vi "RVHR Run MetaInfo.vi"(8 "error in (no error)":errorcluster, 10 "Run Info":T1 {"Date" format="%<%d/%m/%Y>T"}) -> (0 "error out":errorcluster, 2 "RVHR Info File":T2, 3 "Cancel?":bool)   [LabVIEW 2024]
uses:
  Buttons/OK.ctl
  Buttons/Cancel.ctl
  Controls/Sum File Cluster (RCA).ctl
  Controls/File Information CLuster.ctl
  Controls/Run Description.ctl
  Controls/Run information (YRCA).ctl
  Controls/System information (YRCA - Truncate).ctl
panel:
  in  "OK Button":T7
  in  "Cancel Button":T8
  in  "Ref Profile":string caption="Ref Profile:"
  in  "Company":string caption="Company:"
  in  "Location":string caption="Location:"
  in  "Operator":string caption="Operator:"
  in  "Date":timestamp caption="Date:" format="%<%d/%m/%Y>T"
  in  "Run End":dbl caption="Run End:" format="%.3f km"
  in  "Run Start":dbl caption="Run Start:" format="%.3f km"
  in  "Notes":string caption="Notes:"
  # "Enter Information for the Run:"
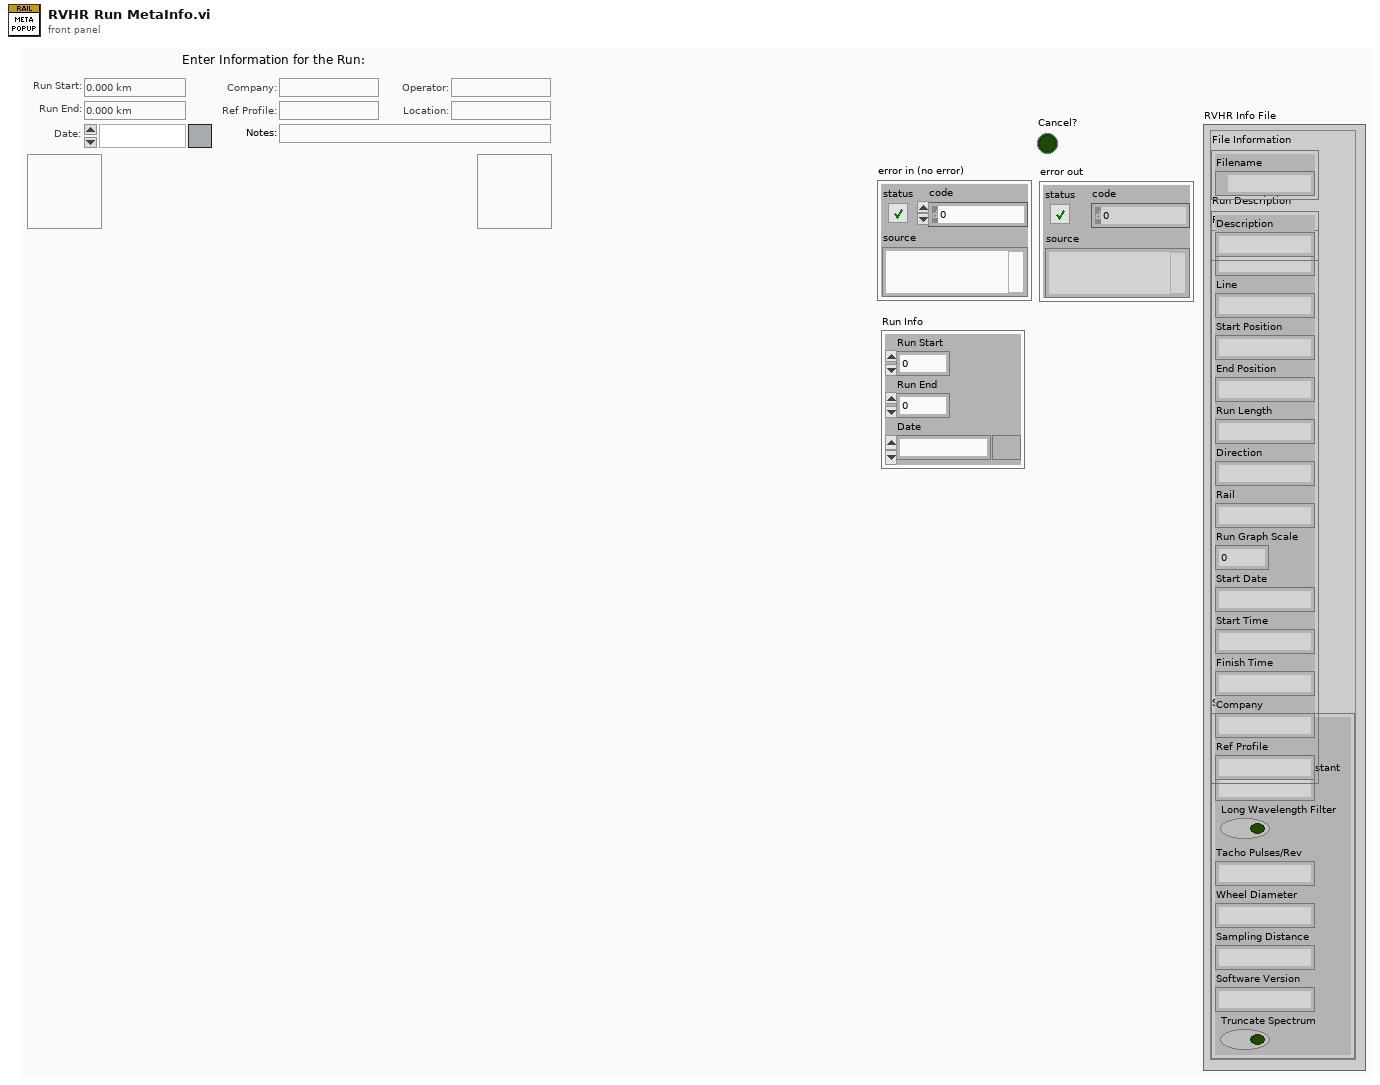
[diagram p1: front panel]
types:
  T1 = cluster{"Run Start":dbl, "Run End":dbl, "Date":timestamp}
  T2 = typedef "Sum File Cluster (RCA).ctl" = cluster{"File Information":T3, "Run Description":T4, "Run Information":T5, "System Information":T6}
  T3 = typedef "File Information CLuster.ctl" = cluster{"Filename":path}
  T4 = typedef "Run Description.ctl" = cluster{"Description":string}
  T5 = typedef "Run information (YRCA).ctl" = cluster{"Operator":string, "Line":string, "Start Position":string, "End Position":string, "Run Length":string, "Direction":string, "Rail":string, "Run Graph Scale":u16, "Start Date":string, "Start Time":string, "Finish Time":string, "Company":string, "Ref Profile":string}
  T6 = typedef "System information (YRCA - Truncate).ctl" = cluster{"Sensor Calibration":string, "Integrator Time Constant":string, "Long Wavelength Filter":bool, "Tacho Pulses/Rev":string, "Wheel Diameter":string, "Sampling Distance":string, "Software Version":string, "Truncate Spectrum":bool}
  T7 = typedef "OK.ctl" = bool
  T8 = typedef "Cancel.ctl" = bool
  T9 = enum8{"Enabled", "Disabled", "Disabled and Grayed Out"}
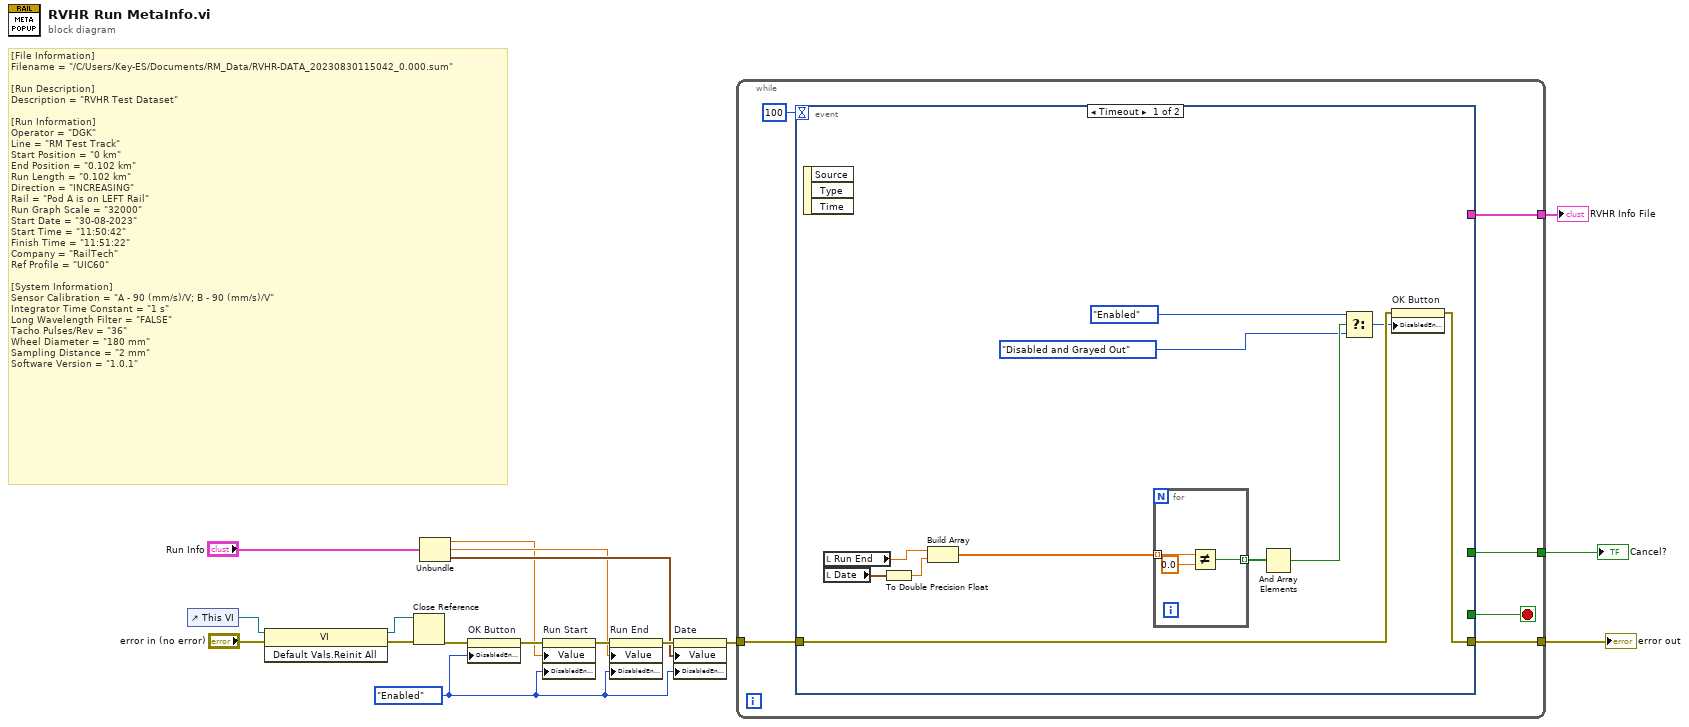
[diagram p0: block diagram]
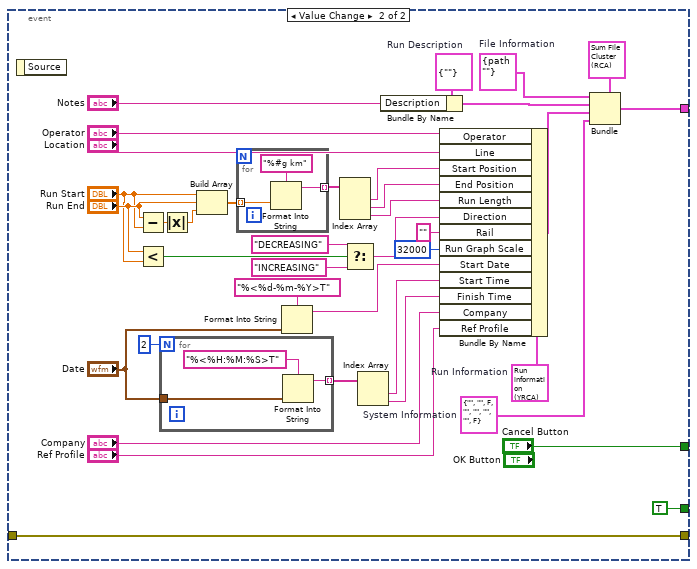
[diagram p2: hidden frame]
diagram:
  w1 = T9."Enabled" ("Disabled")
  # "[File Information]\nFilename = \"/C/Users/Key-ES/Documents/RM_Data/RVHR-DATA_20230830115042_0.000.sum\"\n\n[Run Description]\nDescription = \"RVHR Test Dataset\"\n\n[Run Information]\nOperator = \"DGK\"\nLine = \"RM Test Track\"\nStart Position = \"0 km\"\nEnd Position = \"0.102 km\"\nRun Length = \"0.102 km\"\nDirection = \"INCREASING\"\nRail = \"Pod A is on LEFT Rail\"\nRun Graph Scale = \"32000\"\nStart Date = \"30-08-2023\"\nStart Time = \"11:50:42\"\nFinish Time = \"11:51:22\"\nCompany = \"RailTech\"\nRef Profile = \"UIC60\"\n\n[System Information]\nSensor Calibration = \"A - 90 (mm/s)/V; B - 90 (mm/s)/V\"\nIntegrator Time Constant = \"1 s\"\nLong Wavelength Filter = \"FALSE\"\nTacho Pulses/Rev = \"36\"\nWheel Diameter = \"180 mm\"\nSampling Distance = \"2 mm\"\nSoftware Version = \"1.0.1\""
  n1 = control-ref of="This VI"() -> (w13:refnum<vi>)
  n2 = invoke class="VI" method="Default Vals.Reinit All"(reference=w13, error in="error in (no error)") -> (reference out=w12:refnum<vi>, error out=w14:errorcluster)  [unwired: 1 in, 1 out]
  n3 = Close Reference(reference=w12, error in (no error)=w14) -> (error out=w11:errorcluster)
  n4 = Unbundle("Run Info") -> ("Run Start"=w2:dbl, "Run End"=w3:dbl, "Date"=w4:timestamp)
  n5 = property on="OK Button" class="Bool"(error in=w11, "DisabledEnum"=w1) -> (error out=w6:errorcluster)  [unwired: 1 in, 1 out]
  n6 = property on="Run Start" class="DigNum (strict)"(error in=w6, "Value"=w2, "DisabledEnum"=w1) -> (error out=w9:errorcluster)  [unwired: 1 in, 1 out]
  n7 = property on="Run End" class="DigNum (strict)"(error in=w9, "Value"=w3, "DisabledEnum"=w1) -> (error out=w8:errorcluster)  [unwired: 1 in, 1 out]
  n8 = property on="Date" class="AbsTime (strict)"(error in=w8, "Value"=w4, "DisabledEnum"=w1) -> (error out=w7:errorcluster)  [unwired: 1 in, 1 out]
  n9 = while {
    tunnel: w7 -> [w23]
    tunnel: [w22] -> w16
    tunnel: [w21] -> w15
    tunnel: [w18] -> w10
    stop <- w20 stop-if-true
    n10 = event shown="[0] Timeout" {
      selector: _ -> [_ _]
      dyn-events: _ -> [_ _]
      timeout: 100 -> [_ _]
      tunnel: w23 -> [w29 w75]
      tunnel: [w28 w75] -> w22
      tunnel: [_ "Cancel Button"] -> w21
      tunnel: [_ TRUE] -> w20
      tunnel: [_ w38] -> w18
      event Timeout {
        n11 = event-data() -> ()  [unwired: 1 in, 3 out]
        n12 = local read "Run End"() -> (w33:dbl)
        n13 = local read "Date"() -> (w32:timestamp)
        n14 = To Double Precision Float(number=w32) -> (double precision float=w31:dbl)
        n15 = Build Array(w33, w31) -> (w34:dbl[])
        n16 = for {
          tunnel: w34 -> [w36] mode=indexing
          tunnel: [w35] -> w30 mode=indexing
          n17 = Not Equal?(x=w36, y=0.0) -> (x != y?=w35:bool)
        }
        n18 = And Array Elements(Boolean array=w30) -> (logical AND=w27:bool)
        n19 = Select(t=T9."Enabled", s=w27, f=T9."Disabled and Grayed Out" ("Disabled")) -> (s? t:f=w25:T9)
        n20 = property on="OK Button" class="Bool"(error in=w29, "DisabledEnum"=w25) -> (error out=w28:errorcluster)  [unwired: 1 in, 1 out]
      }
      event Value Change {
        w64 = T6 {"Sensor Calibration"="", "Integrator Time Constant"="", "Long Wavelength Filter"=FALSE, "Tacho Pulses/Rev"="", "Wheel Diameter"="", "Sampling Distance"="", "Software Version"="", "Truncate Spectrum"=FALSE}  # System Information
        w67 = T5 {"Operator"="", "Line"="", "Start Position"="", "End Position"="", "Run Length"="", "Direction"="", "Rail"="", "Run Graph Scale"=0, "Start Date"="", "Start Time"="", "Finish Time"="", "Company"="", "Ref Profile"=""}  # Run Information
        w69 = T3 {"Filename"=path ""}  # File Information
        w71 = T4 {"Description"=""}  # Run Description
        n21 = event-data() -> ()  [unwired: 1 in, 1 out]
        n22 = Subtract(x="Run End", y="Run Start") -> (x-y=w57:dbl)
        n23 = Less?(x="Run End", y="Run Start") -> (x < y?=w46:bool)
        n24 = for {
          N: 2 -> [_]
          tunnel: "Date" -> [w77]
          tunnel: [w76] -> w45 mode=indexing
          n25 = Format Into String(format string="%<%H:%M:%S>T", w77) -> (resulting string=w76:string)  [unwired: 2 in, 1 out]
        }
        n26 = Absolute Value(x=w57) -> (abs(x)=w58:dbl)
        n27 = Build Array("Run Start", "Run End", w58) -> (w56:dbl[])
        n28 = for {
          tunnel: w56 -> [w81] mode=indexing
          tunnel: [w79] -> w55 mode=indexing
          n29 = Format Into String(format string="%#g km", w81) -> (resulting string=w79:string)  [unwired: 2 in, 1 out]
        }
        n30 = Format Into String(format string="%<%d-%m-%Y>T", "Date") -> (resulting string=w41:string)  [unwired: 2 in, 1 out]
        n31 = Index Array(array=w55) -> (element #1=w54:string, element #2=w53:string, element #3=w52:string)  [unwired: 3 in]
        n32 = Select(t="DECREASING", s=w46, f="INCREASING") -> (s? t:f=w49:string)
        n33 = Index Array(array=w45) -> (element #1=w40:string, element #2=w39:string)  [unwired: 2 in]
        n34 = Bundle By Name(cluster=w71, "Description"="Notes") -> (w68:T4)
        n35 = Bundle By Name(cluster=w67, "Operator"="Operator", "Line"="Location", "Start Position"=w54, "End Position"=w53, "Run Length"=w52, "Direction"=w49, "Rail"="", "Run Graph Scale"=u16 32000, "Start Date"=w41, "Start Time"=w40, "Finish Time"=w39, "Company"="Company", "Ref Profile"="Ref Profile") -> (w65:T5)
        n36 = Bundle(cluster=T2 {"File Information"={"Filename"=path ""}, "Run Description"={"Description"=""}, "Run Information"={"Operator"="", "Line"="", "Start Position"="", "End Position"="", "Run Length"="", "Direction"="", "Rail"="", "Run Graph Scale"=0, "Start Date"="", "Start Time"="", "Finish Time"="", "Company"="", "Ref Profile"=""}, "System Information"={"Sensor Calibration"="", "Integrator Time Constant"="", "Long Wavelength Filter"=FALSE, "Tacho Pulses/Rev"="", "Wheel Diameter"="", "Sampling Distance"="", "Software Version"="", "Truncate Spectrum"=FALSE}} ("output cluster"), "File Information"=w69, "Run Description"=w68, "Run Information"=w65, "System Information"=w64) -> (w38:T2)
      }
    }
  }
  "Cancel?" <- w15
  "error out" <- w16
  "RVHR Info File" <- w10
